vi "Decode Car State.vi"(11 "Numeric":u8) -> (3 "Car State":T1(ring))   [LabVIEW 2014]
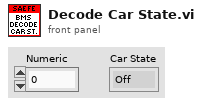
[diagram p1: front panel]
types:
  T1 = enum16{"Off", "On, Not Charging", "Charging", "Charging Finished", "Charging Error"}
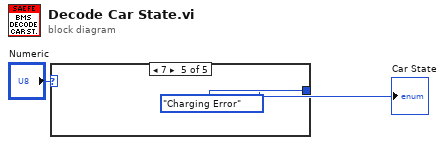
[diagram p0: block diagram]
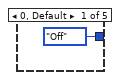
[diagram p2: hidden frame]
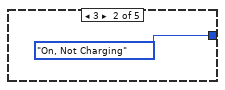
[diagram p3: hidden frame]
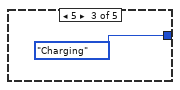
[diagram p4: hidden frame]
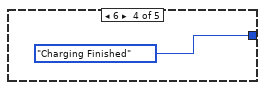
[diagram p5: hidden frame]
diagram:
  n1 = case shown="7" "Numeric" {
    tunnel: [T1."Off" ("Car State") T1."On, Not Charging" ("Car State") T1."Charging" ("Car State") T1."Charging Finished" ("Car State") T1."Charging Error" ("Car State")] -> w1
    frame 0, Default {
    }
    frame 3 {
    }
    frame 5 {
    }
    frame 6 {
    }
    frame 7 {
    }
  }
  "Car State" <- w1
